vi "Core.vi"(8 "Negative Fit":refnum<class "Sinusoidal Fit.lvclass">, 9 "Positive Fit":refnum<class "Sinusoidal Fit.lvclass">, 11 "Event Registration Refnum":refnum<event-registration>) -> ()   [LabVIEW 2016, in "Halfwave Fit Display.lvclass"]
uses:
  Halfwave Fit Display.lvclass
  gain and phase/Typedef - Sinusoidal Fit Coefficients.ctl
  Sinusoidal Fit/Sinusoidal Fit.lvclass
  gain and phase/Typedef - Gain and Phase.ctl
panel:
  out "Positive Halfwave":T1 {"Phase SD" format="%.1f"; "Phase" format="%.1f"; "Gain SD" format="%.2f"; "Gain" format="%.2f"}
  out "Negative Halfwave":T1 {"Phase SD" format="%.1f"; "Phase" format="%.1f"; "Gain SD" format="%.2f"; "Gain" format="%.2f"}
  out "Coefficients":T2 {"Freq" format="%#.2f"; "Offset" format="%.3f"; "Gain" format="%.2f"; "Phase" format="%.1f"}
  in  "Response":T2 {"Freq" format="%#.2f"; "Offset" format="%.3f"; "Gain" format="%.2f"; "Phase" format="%.1f"}
  out "Coefficients 2":T2 {"Freq" format="%#.2f"; "Offset" format="%.3f"; "Gain" format="%.2f"; "Phase" format="%.1f"}
  in  "Coefficients 3":T2 {"Freq" format="%#.2f"; "Offset" format="%.3f"; "Gain" format="%.2f"; "Phase" format="%.1f"}
  # "Gain:"
  # "+/-"
  # "Phase:"
  # "+/-"
  # "Gain:"
  # "+/-"
  # "Phase:"
  # "+/-"
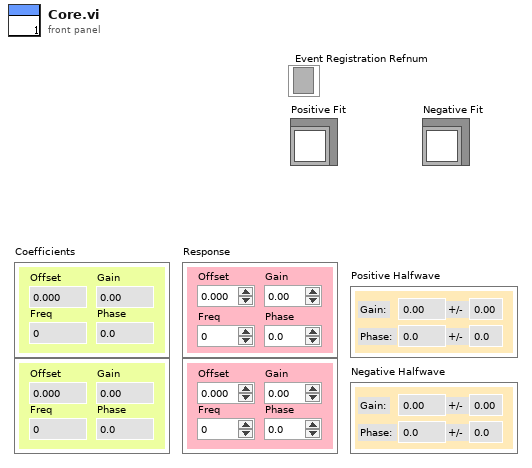
[diagram p1: front panel]
types:
  T1 = typedef "Typedef - Gain and Phase.ctl" = cluster{"Gain":dbl, "Gain SD":dbl, "Phase":dbl, "Phase SD":dbl}
  T2 = typedef "Typedef - Sinusoidal Fit Coefficients.ctl" = cluster{"Offset":dbl, "Gain":dbl, "Phase":dbl, "Freq":dbl}
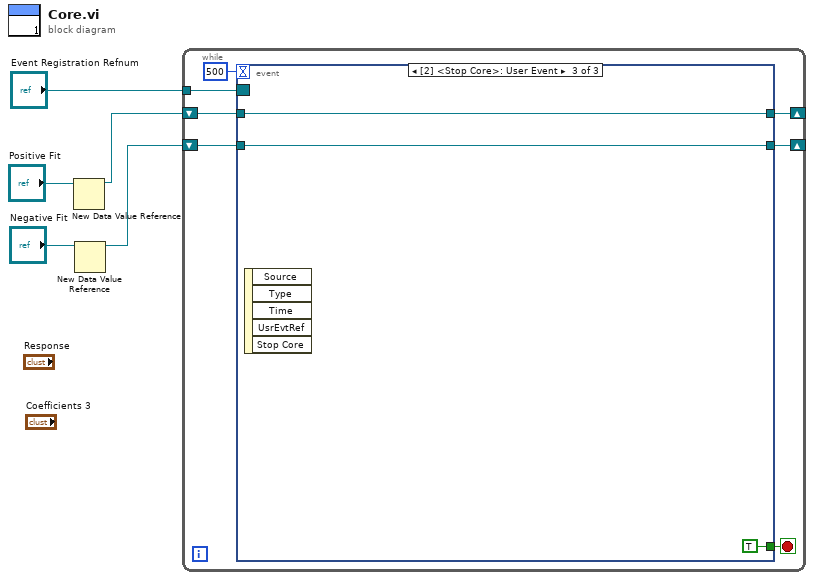
[diagram p0: block diagram]
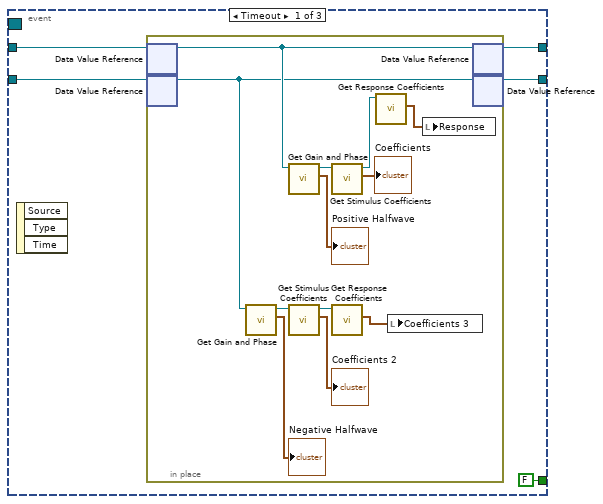
[diagram p2: hidden frame]
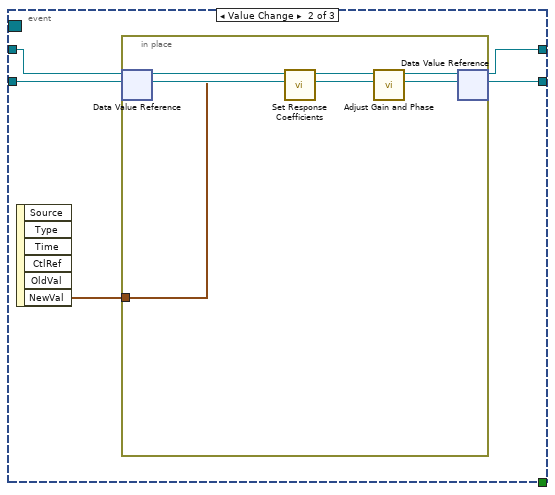
[diagram p3: hidden frame]
diagram:
  n1 = New Data Value Reference(data value="Positive Fit") -> (data value reference=w2:refnum<data-value>)  [unwired: 1 in, 1 out]
  n2 = New Data Value Reference(data value="Negative Fit") -> (data value reference=w1:refnum<data-value>)  [unwired: 1 in, 1 out]
  n3 = while {
    tunnel: "Event Registration Refnum" -> [w11]
    shift-right: [w7] -> _
    shift-left: w2 -> [w9]
    shift-right: [w6] -> _
    shift-left: w1 -> [w8]
    stop <- w12 stop-if-true
    n4 = event shown="[2] <Stop Core>: User Event" {
      selector: w11 -> [_ _ _]
      dyn-events: _ -> [_ _ _]
      timeout: 500 -> [_ _ _]
      tunnel: [FALSE _ TRUE] -> w12
      tunnel: w9 -> [w16 w33 w39]
      tunnel: w8 -> [w15 w30 w38]
      tunnel: [w14 w32 w39] -> w7
      tunnel: [w13 w30 w38] -> w6
      event Timeout {
        n5 = event-data() -> ()  [unwired: 1 in, 3 out]
        n6 = in-place {
          n7 = in-place-dvr #1(w16) -> (w21:refnum<class "Sinusoidal Fit.lvclass">)  [unwired: 1 out]
          n8 = in-place-dvr #2(w15) -> (w20:refnum<class "Sinusoidal Fit.lvclass">)  [unwired: 1 out]
          n9 = call-dynamic "Get Gain and Phase.vi"("Sinusoidal Fit in"=w20) -> ("Gain and Phase"=→"Negative Halfwave":T1, "Sinusoidal Fit out"=w27:refnum<class "Sinusoidal Fit.lvclass">)  [unwired: 8 in, 1 out]
          n10 = call-dynamic "Get Gain and Phase.vi"("Sinusoidal Fit in"=w21) -> ("Gain and Phase"=→"Positive Halfwave":T1, "Sinusoidal Fit out"=w24:refnum<class "Sinusoidal Fit.lvclass">)  [unwired: 8 in, 1 out]
          n11 = call-dynamic "Get Stimulus Coefficients.vi"("Sinusoidal Fit in"=w27) -> ("Coefficients"=→"Coefficients 2":T2, "Sinusoidal Fit out"=w28:refnum<class "Sinusoidal Fit.lvclass">)  [unwired: 8 in, 1 out]
          n12 = call-dynamic "Get Stimulus Coefficients.vi"("Sinusoidal Fit in"=w24) -> ("Coefficients"=→"Coefficients":T2, "Sinusoidal Fit out"=w25:refnum<class "Sinusoidal Fit.lvclass">)  [unwired: 8 in, 1 out]
          n13 = call-dynamic "Get Response Coefficients.vi"("Sinusoidal Fit in"=w28) -> ("Coefficients"=w18:T2)  [unwired: 8 in, 2 out]
          n14 = call-dynamic "Get Response Coefficients.vi"("Sinusoidal Fit in"=w25) -> ("Coefficients"=w19:T2)  [unwired: 8 in, 2 out]
          n15 = local write "Coefficients 3"(w18) -> ()
          n16 = local write "Response"(w19) -> ()
          n17 = in-place-dvr #1(w21) -> (w14:refnum<data-value>)  [unwired: 1 out]
          n18 = in-place-dvr #2(w20) -> (w13:refnum<data-value>)  [unwired: 1 out]
        }
      }
      event Value Change {
        n19 = event-data() -> ("NewVal"=w31:T2)  [unwired: 1 in, 5 out]
        n20 = in-place {
          in-place-border: w31 -> [w36]
          n21 = in-place-dvr #3(w33) -> (w37:refnum<class "Sinusoidal Fit.lvclass">)  [unwired: 1 out]
          n22 = call-dynamic "Set Response Coefficients.vi"("Coefficients"=w36, "Sinusoidal Fit in"=w37) -> ("Sinusoidal Fit out"=w35:refnum<class "Sinusoidal Fit.lvclass">)  [unwired: 8 in, 1 out]
          n23 = call-dynamic "Adjust Gain and Phase.vi"("Sinusoidal Fit in"=w35) -> ("Sinusoidal Fit out"=w34:refnum<class "Sinusoidal Fit.lvclass">)  [unwired: 9 in, 1 out]
          n24 = in-place-dvr #3(w34) -> (w32:refnum<data-value>)  [unwired: 1 out]
        }
      }
      event User Event {
        n25 = event-data() -> ()  [unwired: 1 in, 5 out]
      }
    }
  }
